vi "SMTP Email MIME Text Content-Type.vi"(4 "translit":string, 5 "name":string, 6 "character set":string) -> (0 "MIME content-type":string)   [LabVIEW 2012, in "NewNI_SMTPEmail.lvlib"]
uses:
  NewNI_SMTPEmail.lvlib
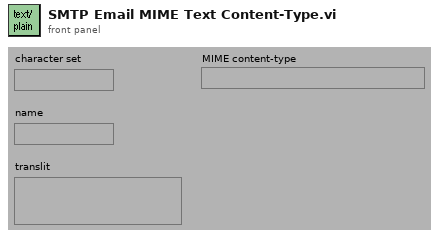
[diagram p1: front panel]
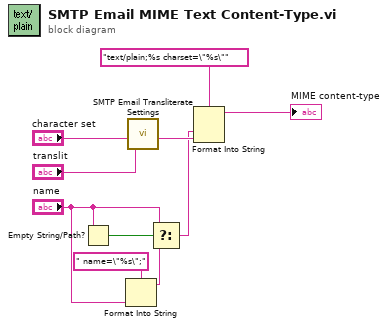
[diagram p0: block diagram]
diagram:
  n1 = Empty String/Path?(string/path="name") -> (empty?=w6:bool)
  n2 = Format Into String(format string=" name=\"%s\";", "name") -> (resulting string=w4:string)  [unwired: 2 in, 1 out]
  n3 = call "SMTP Email Transliterate Settings.vi"("transliteration"="translit", "character set"="character set") -> ("charset out"=w8:string)  [unwired: 5 out]
  n4 = Select(t="name", s=w6, f=w4) -> (s? t:f=w3:string)
  n5 = Format Into String(format string="text/plain;%s charset=\"%s\"", w3, w8) -> (resulting string=→"MIME content-type":string)  [unwired: 2 in, 1 out]
